vi "Get Autorange Bereiche.vi"(8 "error in (no error)":errorcluster caption="Fehler (Eingang, kein Fehler)", 11 "Gaskomponente":T2) -> (0 "error out":errorcluster caption="Fehler (Ausgang)", 2 "Autorange Bereiche":T1[](array[typedef]), 3 "Autorange Bereiche":T2[](array[typedef]))   [LabVIEW 2020, in "Linearisierung v2.lvlib"]
uses:
  Linearisierung v2.lvlib
  Visualisierungs Elemente/Auswahlfeld.ctl
  Visualisierungs Elemente/String - Ausgabefeld.ctl
  Seiten/FT-IR/FGV FT-IR Gasliste Aktionen.ctl
  <vilib>/regexp/Match Regular Expression.xnode
  Seiten/FT-IR/FT-IR.lvlib
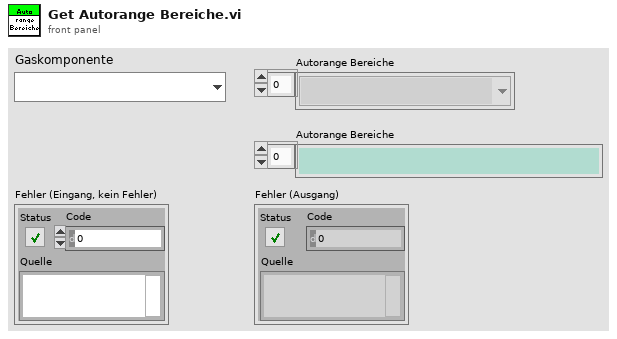
[diagram p1: front panel]
types:
  T1 = typedef "String - Ausgabefeld.ctl" = string
  T2 = typedef "Auswahlfeld.ctl" = u16
  T3 = typedef "FT-IR.lvlib/FGV FT-IR Gasliste Aktionen.ctl" = enum16{"lesen", "Gasliste FT-IR", "Gasliste ausgelesen", "laden", "speichern", "löschen"}
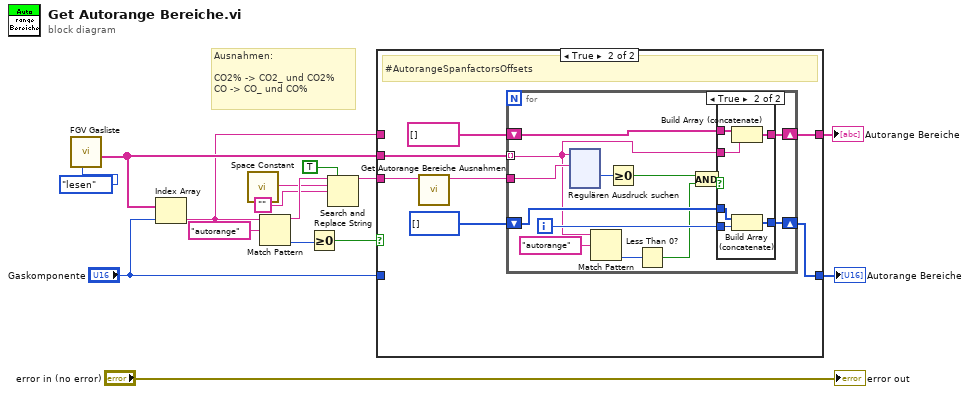
[diagram p0: block diagram]
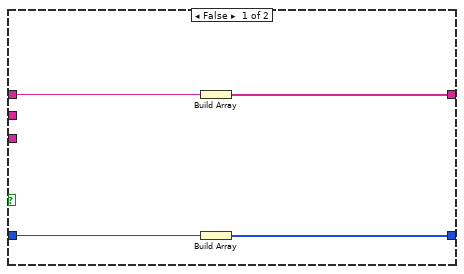
[diagram p2: hidden frame]
diagram:
  # "Ausnahmen:\n\nCO2% -> CO2_ und CO2%\nCO -> CO_ und CO%"
  n1 = call "FGV Gasliste.vi"("Aktionen"=FGV_FT-IR_Gasliste_Aktionen."lesen") -> ("Aktuelle Gasliste gesamt"=w8:T1[])  [unwired: 8 in, 2 out]
  n2 = Index Array(array=w8, index="Gaskomponente") -> (element=w1:T1)
  n3 = call <vilib>:"Space Constant.vi"() -> ("String"=w6:string)
  n4 = Match Pattern(string=w1, regular expression="autorange" ("Regulärer Ausdruck")) -> (before substring=w7:T1, offset past match=w13:i32)  [unwired: 1 in, 2 out]
  n5 = Greater Or Equal To 0?(x=w13) -> (x >= 0?=w12:bool)
  n6 = Search and Replace String(replace all?=TRUE ("Alle ersetzen? (F)"), input string=w7, search string=w6, replace string="") -> (result string=w3:string)  [unwired: 4 in, 3 out]
  n7 = case shown="True" w12 {
    tunnel: "Gaskomponente" -> [w19 _]
    tunnel: [w18 w24] -> w9
    tunnel: w8 -> [_ w26]
    tunnel: w3 -> [_ w21]
    tunnel: [w16 w22] -> w2
    tunnel: w1 -> [w17 _]
    frame False {
      n8 = Build Array(w17) -> (w16:T1[])
      n9 = Build Array(w19) -> (w18:T2[])
    }
    frame True {
      # "#AutorangeSpanfactorsOffsets"
      n10 = call "Get Autorange Bereiche Ausnahmen.vi"("result string (Eingang)"=w21) -> ("result string (Ausgang)"=w20:string)  [unwired: 10 in]
      n11 = for {
        tunnel: w26 -> [w29] mode=indexing
        tunnel: w20 -> [w39]
        shift-right: [w36] -> w24
        shift-left: i32[] [] -> [w35]
        shift-right: [w34] -> w22
        shift-left: T1[] [] -> [w33]
        i -> [w37]
        n12 = xnode "Regulären Ausdruck suchen"("Eingangs-String"=w29, "Regulärer Ausdruck"=w39) -> ("Offset nach Übereinstimmung"=w32:i32)  [unwired: 4 in, 4 out]
        n13 = Match Pattern(string=w29, regular expression="autorange" ("Regulärer Ausdruck")) -> (offset past match=w28:i32)  [unwired: 1 in, 3 out]
        n14 = Greater Or Equal To 0?(x=w32) -> (x >= 0?=w38:bool)
        n15 = Less Than 0?(x=w28) -> (x < 0?=w27:bool)
        n16 = And(x=w38, y=w27) -> (x .and. y?=w31:bool)
        n17 = case shown="True" w31 {
          tunnel: w37 -> [_ w161]
          tunnel: [w155 w160] -> w36
          tunnel: w35 -> [w155 w159]
          tunnel: [w154 w158] -> w34
          tunnel: w33 -> [w154 w157]
          tunnel: w29 -> [_ w156]
          frame False {
          }
          frame True {
            n18 = Build Array (concatenate)(w157, w156) -> (w158:T1[])
            n19 = Build Array (concatenate)(w159, w161) -> (w160:i32[])
          }
        }
      }
    }
  }
  "Autorange Bereiche" <- w9
  "Autorange Bereiche" <- w2
  "error out" <- "error in (no error)"
